vi "mupExpr Demo3.vi"() -> ()   [LabVIEW 2015]
uses:
  mupExpr/mupExpr.lvclass/mupExpr.ctl
  mupExpr/SetVarVal.vi
  mupLib/mupEvalMulti.vi
  mupLib/mupSetVarValue.vi
  mupLib/mupCheckError.vi
  mupLib/mupLibPath.vi
  <vilib>/Utility/error.llb/Error Cluster From Error Code.vi
  mupExpr/mupExpr.lvclass
panel:
  out "error out":errorcluster
  out "Results":dbl[](array[numeric]) format="%#_13g"
  out "Variable Names":string[](array[string])
  in  "Expression":string="a*x+b,\na,\n3*x+a"
  in  "varValues":dbl[](array[numeric])=[1.0, 1.0, 5.0] format="%#_13g"
  # "Multiple variables, Multiple expressions"
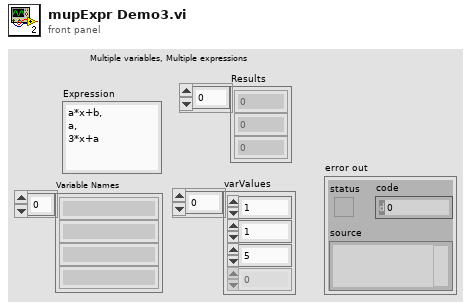
[diagram p1: front panel]
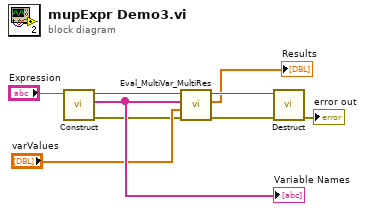
[diagram p0: block diagram]
diagram:
  n1 = call "Construct.vi"("Expression"="Expression") -> ("error out"=w4:errorcluster, "Variable Names"=w6:string[], "mupExpr out"=w3:refnum<data-value>)  [unwired: 8 in]
  "Variable Names" <- w6
  n2 = call "Eval_MultiVar_MultiRes.vi"("error in (no error)"=w4, "varValues"="varValues", "varNames"=w6, "mupExpr in"=w3) -> ("error out"=w7:errorcluster, "Results"=→"Results":dbl[], "mupExpr out"=w8:refnum<data-value>)  [unwired: 5 in]
  n3 = call "Destruct.vi"("error in (no error)"=w7, "mupExpr in"=w8) -> ("error out"=→"error out":errorcluster)  [unwired: 9 in]
